vi "Create Connection.vi"(8 "error in (no error)":errorcluster, 11 "IConnectionFactory in":refnum<class "IConnectionFactory.lvclass">) -> (0 "error out":errorcluster, 2 "Connection":refnum<class "IConnection.lvclass">, 3 "IConnectionFactory out":refnum<class "IConnectionFactory.lvclass">)   [LabVIEW 2019, in "IConnectionFactory.lvclass"]
uses:
  <vilib>/gpm_packages/@cs/Network-interface/Source/IConnectionFactory/IConnectionFactory.lvclass
  <vilib>/gpm_packages/@cs/Network-interface/Source/Connection Reference/IConnection/IConnection.lvclass
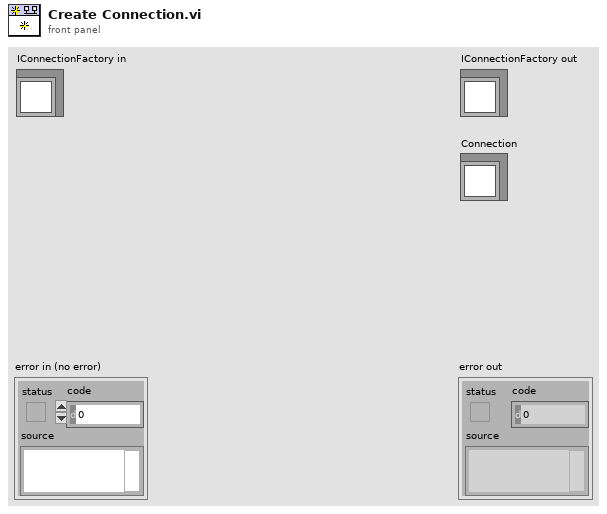
[diagram p1: front panel]
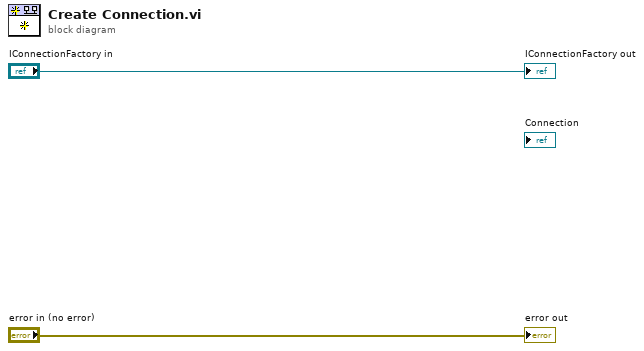
[diagram p0: block diagram]
diagram:
  "error out" <- "error in (no error)"
  "IConnectionFactory out" <- "IConnectionFactory in"
